vi "Load Section - Logging.vi"(8 "error in (no error)":errorcluster, 11 "JSON string":string) -> (0 "error out":errorcluster, 3 "Class data":refnum<class "Settings Service.lvclass">)   [LabVIEW 2026, in "Settings Service.lvclass"]
uses:
  Settings Service.lvclass
  Settings Service.lvclass/Settings Service.ctl
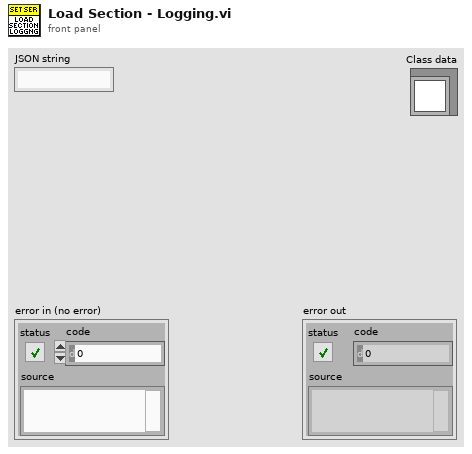
[diagram p1: front panel]
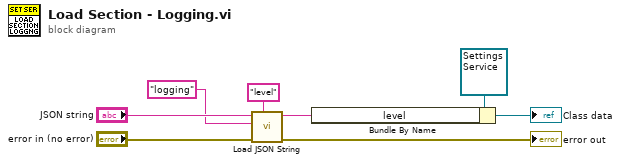
[diagram p0: block diagram]
diagram:
  n1 = call "Load JSON String.vi"("Element"="level", "error in (no error)"="error in (no error)", "Section"="logging", "JSON string"="JSON string") -> ("error out"=→"error out":errorcluster, "value"=w2:string)  [unwired: 6 in]
  n2 = Bundle By Name(cluster=refnum<class "Settings Service.lvclass"> refnum ("Settings Service.lvclass"), "level"=w2) -> (→"Class data":refnum<class "Settings Service.lvclass">)
